vi "Read.vi"(8 "error in (no error)":errorcluster, 9 "Starting independent variable":dbl, 10 "Current independent variable":dbl, 11 "multimeter reader in":refnum<class "multimeter reader.lvclass">) -> (0 "error out":errorcluster, 2 "Data Channels":T1, 3 "multimeter reader out":refnum<class "multimeter reader.lvclass">)   [LabVIEW 2009, in "multimeter reader.lvclass"]
doc: "Prepare for read, wait the time delay, and take data from up to 4 channels."
uses:
  multimeter reader.lvclass
  Instruments/Utility Classes/Readable/Data Channels.ctl
  Instruments/Utility Classes/Readable/Data Channel.ctl
  Instruments/Utility Classes/Readable/Data Point.ctl
  Instruments/Utility Classes/Readable/Time.ctl
  Instruments/Utility Classes/Readable/X.ctl
  Reader/Reader.lvclass
  Instruments/Utility Classes/Readable/Readable.lvclass
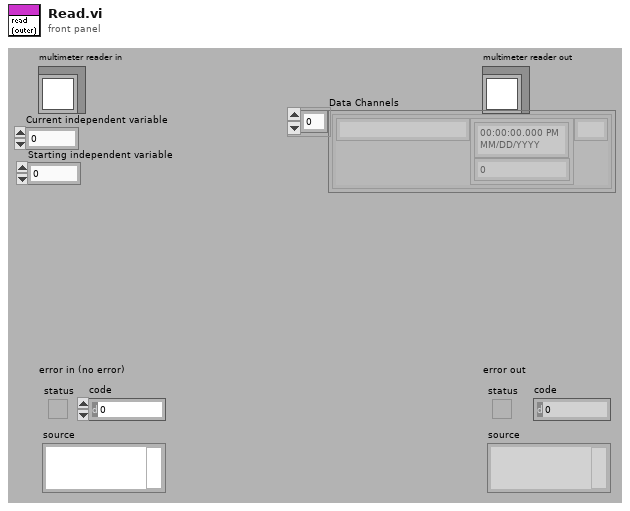
[diagram p1: front panel]
types:
  T1 = typedef "Readable.lvclass/Data Channels.ctl" = T2[]
  T2 = typedef "Readable.lvclass/Data Channel.ctl" = cluster{"Name":string, "Data Point":T3, "Unit":string}
  T3 = typedef "Readable.lvclass/Data Point.ctl" = cluster{"t":T4, "x":T5}
  T4 = typedef "Readable.lvclass/Time.ctl" = timestamp
  T5 = typedef "Readable.lvclass/X.ctl" = dbl
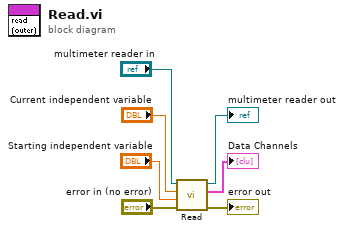
[diagram p0: block diagram]
diagram:
  n1 = call-parent "Read.vi"("error in (no error)"="error in (no error)", "Starting independent variable"="Starting independent variable", "Current independent variable"="Current independent variable", "Reader in"="multimeter reader in") -> ("error out"=→"error out":errorcluster, "Data Channels"=→"Data Channels":T1, "Reader out"=→"multimeter reader out":refnum<class "multimeter reader.lvclass">)  [unwired: 5 in]
